vi "Reference.vi"(7 "Action":enum16{"Get", "Close"}(ring), 8 "error in (no error)":errorcluster) -> (0 "error out":errorcluster, 3 "Refnum out":T1)   [LabVIEW 2020, in "Configuration Manager.lvclass"]
uses:
  Configuration Manager.lvclass
  <vilib>/Utility/config.llb/Config Data RefNum.ctl
  Configuration Manager.lvclass/Configuration Manager.ctl
  <vilib>/Utility/config.llb/NI_LVConfig.lvlib
  <vilib>/Utility/sysdir.llb/System Directory Type.ctl
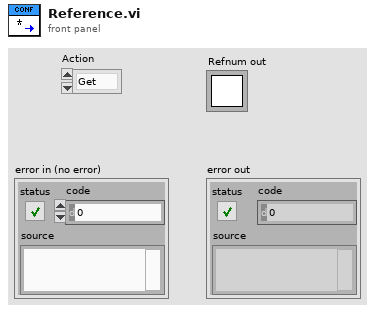
[diagram p1: front panel]
types:
  T1 = typedef "NI_LVConfig.lvlib/Config Data RefNum.ctl" = refnum<k1>
  T2 = typedef "System Directory Type.ctl" = i32
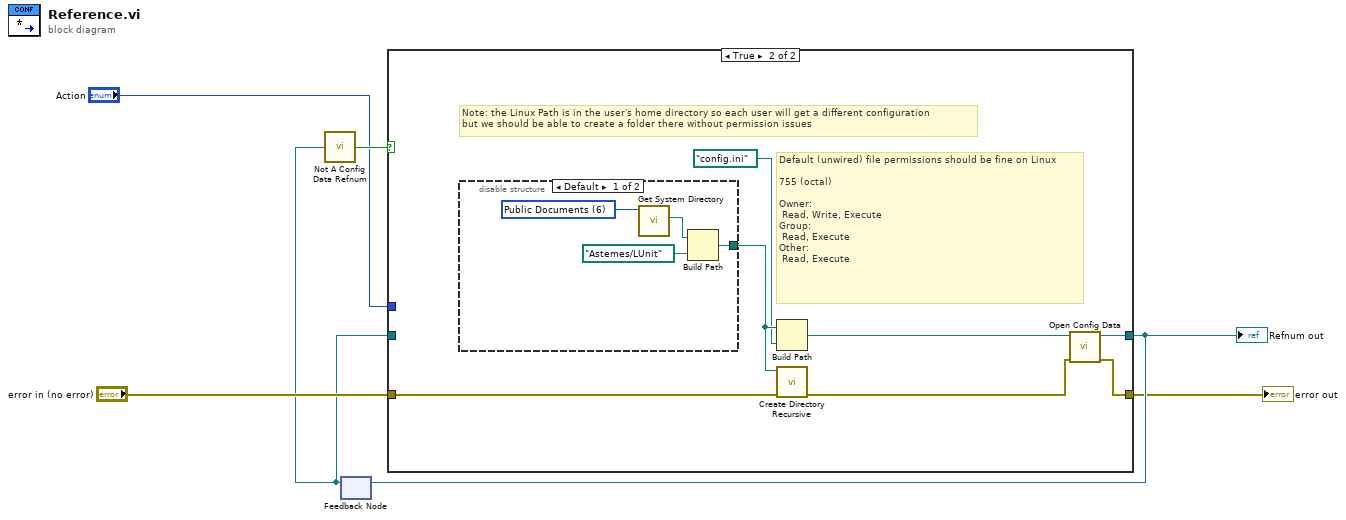
[diagram p0: block diagram]
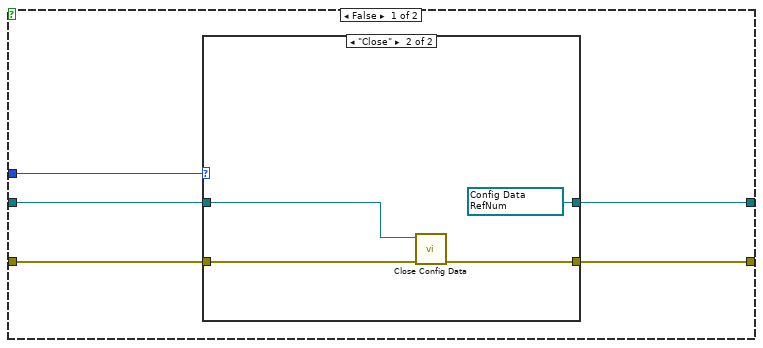
[diagram p2: hidden frame]
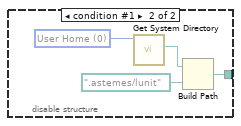
[diagram p4: hidden frame]
diagram:
  n1 = feedback #1() -> (w3:T1)  [unwired: 1 in]
  n2 = call <vilib>:"Not A Config Data Refnum.vi"("refnum"=w3) -> ("not a config data refnum"=w2:bool)
  n3 = case shown="True" w2 {
    tunnel: [w7 w24] -> w6
    tunnel: "error in (no error)" -> [w11 w21]
    tunnel: [w10 w20] -> w5
    tunnel: w3 -> [w8 _]
    tunnel: "Action" -> [w9 _]
    frame False {
      n4 = case shown="\"Close\"" w9 {
        tunnel: w11 -> [w13 w17]
        tunnel: [w13 w16] -> w10
        tunnel: w8 -> [w12 w15]
        tunnel: [w12 w14] -> w7
        frame "Get" {
        }
        frame "Close" {
          w14 = T1 refnum items=["config data"] ("refnum")
          n5 = call <vilib>:"Close Config Data.vi"("error in (no error)"=w17, "refnum"=w15) -> ("error out"=w16:errorcluster)  [unwired: 8 in, 1 out]
        }
      }
    }
    frame True {
      # "Note: the Linux Path is in the user's home directory so each user will get a different configuration \nbut we should be able to create a folder there without permission issues"
      # "Default (unwired) file permissions should be fine on Linux\n\n755 (octal) \n\nOwner:\n Read, Write, Execute\nGroup:\n Read, Execute\nOther:\n Read, Execute"
      n6 = disable-structure shown="Default" {
        disable-tunnel: [w28 w29] -> w19
        frame condition #0 (active) {
          w27 = T2 6 items=["User Home"=0, "User Desktop"=1, "User Documents"=2, "User Application Data"=3, "User Preferences"=4, "User Temporary"=5, "Public Documents"=6, "Public Application Data"=7, "Public Preferences"=8, "Public Cache"=13, "System Core Libraries"=9, "System Installed Libraries"=10, "Application Files"=11, "Boot Volume Root"=12] ("system directory type")
          n7 = call <vilib>:"Get System Directory.vi"("system directory type"=w27) -> ("system directory"=w25:path)  [unwired: 10 in]
          n8 = Build Path(base path=w25, name or relative path=path "Astemes/LUnit") -> (appended path=w28:path)
        }
        frame condition #1 {
          w32 = T2 0 items=["User Home"=0, "User Desktop"=1, "User Documents"=2, "User Application Data"=3, "User Preferences"=4, "User Temporary"=5, "Public Documents"=6, "Public Application Data"=7, "Public Preferences"=8, "Public Cache"=13, "System Core Libraries"=9, "System Installed Libraries"=10, "Application Files"=11, "Boot Volume Root"=12] ("system directory type")
          n9 = call <vilib>:"Get System Directory.vi"("system directory type"=w32) -> ("system directory"=w30:path)  [unwired: 10 in]
          n10 = Build Path(base path=w30, name or relative path=path ".astemes/lunit") -> (appended path=w29:path)
        }
      }
      n11 = Build Path(base path=w19, name or relative path=path "config.ini") -> (appended path=w23:path)
      n12 = call <vilib>:"Create Directory Recursive.vi"("error in (no error)"=w21, "directory"=w19) -> ("error out"=w22:errorcluster)  [unwired: 3 in, 2 out]
      n13 = call <vilib>:"Open Config Data.vi"("error in (no error)"=w22, "configuration file path"=w23) -> ("error out"=w20:errorcluster, "refnum"=w24:T1)  [unwired: 7 in, 1 out]
    }
  }
  "Refnum out" <- w6
  "error out" <- w5
  n14 = feedback-in #1(w6) -> ()
